vi "initialize.vi"(0 "HGF_TaskDFSM":refnum<class "HGF_TaskDFSM.lvclass">, 3 "initializationData":variant, 5 "error in (no error)":errorcluster, 7 "binaryString":string, 8 "I8 Array":i8[](array[numeric]), 9 "prependSize? (T)":bool, 11 "byteOrder (0:big-endian, network order)":T1(ring)) -> (14 "dup TaskDFSM":refnum<class "HGF_TaskDFSM.lvclass">, 17 "found?":bool, 19 "error out":errorcluster)   [LabVIEW 2012, in "HGF_DeviceFSM.lvlib" / "HGF_TaskDFSM.lvclass"]
doc: "This is a dynamic dispatch VI to be implemented by child classes to initialize their attributes.\n\n<B>Recommendation:</B> Use Variant for initialization data."
uses:
  HGF_TaskDFSM.lvclass
  HGF_DeviceBaseClasses/HGF_DeviceVisitor/HGF_DeviceVisitor.lvclass
  HGF_BaseClasses/HGF_PVPublisher/HGF_PVPublisher.lvclass
  HGF_BaseClasses/HGF_Factory/HGF_Factory.lvclass
  HGF_BaseClasses/HGF_ThreadTask/HGF_ThreadTask.lvclass
  HGF_TaskDFSM.lvclass/HGF_TaskDFSM.ctl
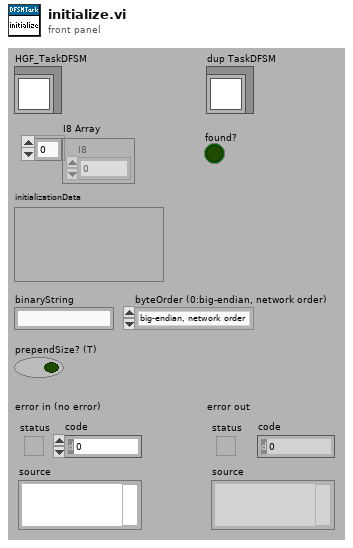
[diagram p1: front panel]
types:
  T1 = enum16{"big-endian, network order", "native, host order", "little-endian"}
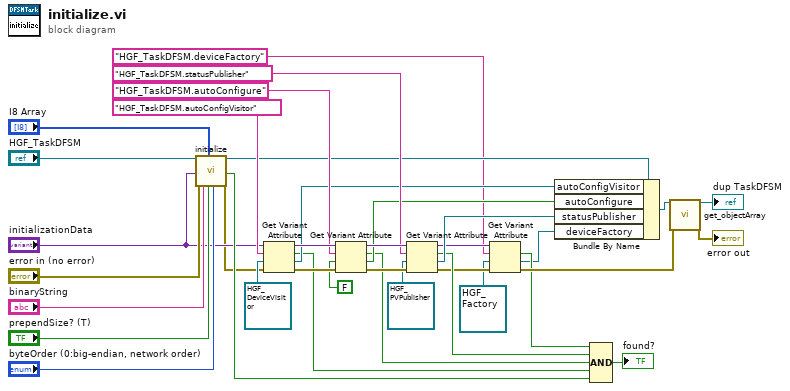
[diagram p0: block diagram]
diagram:
  n1 = call-parent "initialize.vi"("HGF_ThreadTask"="HGF_TaskDFSM", "initializationData"="initializationData", "error in (no error)"="error in (no error)", "binaryString"="binaryString", "I8 Array"="I8 Array", "prependSize? (T)"="prependSize? (T)", "byteOrder (0:big-endian, network order)"="byteOrder (0:big-endian, network order)") -> ("dup HGF_ThreadTask"=w21:refnum<class "HGF_TaskDFSM.lvclass">, "found?"=w17:bool, "error out"=w11:errorcluster)  [unwired: 10 out]
  n2 = Get Variant Attribute(Variant="initializationData", name="HGF_TaskDFSM.autoConfigVisitor", default value (empty Variant)=refnum<class "HGF_DeviceVisitor.lvclass"> refnum ("HGF_DeviceVisitor"), error in=w11) -> (duplicate Variant=w30:variant, found=w16:bool, value=w19:refnum<class "HGF_DeviceVisitor.lvclass">, error out=w31:errorcluster)
  n3 = Get Variant Attribute(Variant=w30, name="HGF_TaskDFSM.autoConfigure", default value (empty Variant)=FALSE ("autoConfigure"), error in=w31) -> (duplicate Variant=w28:variant, found=w15:bool, value=w20:bool, error out=w29:errorcluster)
  n4 = Get Variant Attribute(Variant=w28, name="HGF_TaskDFSM.statusPublisher", default value (empty Variant)=refnum<class "HGF_PVPublisher.lvclass"> refnum ("statusPublisher"), error in=w29) -> (duplicate Variant=w7:variant, found=w14:bool, value=w18:refnum<class "HGF_PVPublisher.lvclass">, error out=w6:errorcluster)
  n5 = Get Variant Attribute(Variant=w7, name="HGF_TaskDFSM.deviceFactory", default value (empty Variant)=refnum<class "HGF_Factory.lvclass"> refnum ("deviceFactory"), error in=w6) -> (found=w2:bool, value=w1:refnum<class "HGF_Factory.lvclass">, error out=w5:errorcluster)  [unwired: 1 out]
  n6 = Bundle By Name(cluster=w21, "autoConfigVisitor"=w19, "autoConfigure"=w20, "statusPublisher"=w18, "deviceFactory"=w1) -> (w10:refnum<class "HGF_TaskDFSM.lvclass">)
  n7 = Compound Arithmetic op=AND(w2, w14, w15, w16, w17) -> (→"found?":bool)
  n8 = call "get_objectArray.vi"("HGF_ThreadTask"=w10, "error in (no error)"=w5) -> ("dup HGF_ThreadTask"=→"dup TaskDFSM":refnum<class "HGF_TaskDFSM.lvclass">, "error out"=→"error out":errorcluster)  [unwired: 16 out]
